vi "testfield.vi"() -> ()   [LabVIEW 2013, in "varilib.lvlib"]
uses:
  varilib.lvlib
panel:
  in  "val 2":dbl format="%_12f"
  out "formatting string":string
  in  "unc-":dbl format="%_2f"
  in  "unc":dbl format="%_2f"
  out "val":dbl format="%_10f"
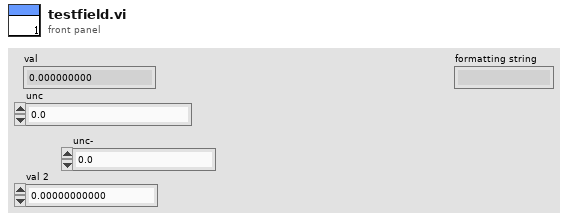
[diagram p1: front panel]
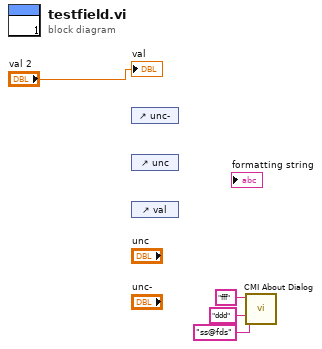
[diagram p0: block diagram]
diagram:
  n1 = control-ref of="unc-"() -> ()  [unwired: 1 out]
  n2 = control-ref of="unc"() -> ()  [unwired: 1 out]
  n3 = control-ref of="val"() -> ()  [unwired: 1 out]
  n4 = call "CMI About Dialog.vi"("E-mail:"="ss@fds", "Author:"="ddd", "Title"="fff" ("title")) -> ()  [unwired: 9 in]
  "val" <- "val 2"
